vi "Compute Fit Curve v4.vi"(0 "X Array in":dbl[](array[numeric]), 1 "# Points":u32, 2 "Use Same Number of Points as Histogram":bool, 5 "Best Fit in":dbl[](array[numeric]), 7 "Y Array in":dbl[](array[numeric]), 11 "Error In":errorcluster, 12 "Fit Model":T2, 13 "Fit Parameters":variant, 14 "Ramp Type":T1 items=["Linear", "Logarithmic"]) -> (4 "Fitted Plot":cluster{"X Array":dbl[], "Y Array":dbl[]}, 6 "Array of Component Plots":cluster{"X Array":dbl[], "Y Array":dbl[]}[](array[cluster]), 8 "Residual Plot":cluster{"X Array":dbl[], "Y Array":dbl[]}, 15 "Error Out":errorcluster)   [LabVIEW 2019]
uses:
  Fit Models.ctl
  Ramp Type.ctl
  Gaussian Fit Results v2.ctl
  Two H-Connected Gaussians Fit Parameters.ctl
  Two H-Connected Asymmetric Gaussians Fit Parameters.ctl
  Asymmetric Gaussian Fit Results v2.ctl
  Two T-Connected Asymmetric Gaussians Fit Parameters.ctl
  Two T-Connected Gaussians Fit Parameters.ctl
  Asymmetric Lorentzian Fit Results v2.ctl
  Gaussian-Lorentzian Fit Results v2.ctl
  Lorentzian-Gaussian Fit Results v2.ctl
  Lorentzian Fit Results v2.ctl
  Single Exponential Fit Parameters v2.ctl
  Double Exponential Fit Parameters v2.ctl
  2D Gaussian ACF Fit Results.ctl
  2D Gaussian + Blinking ACF Fit Results.ctl
  2D Gaussian + Flow ACF Fit Results.ctl
  3D Gaussian ACF Fit Results.ctl
  3D Gaussian + Blinking ACF Fit Results.ctl
  <vilib>/Analysis/NI_AALBase.lvlib
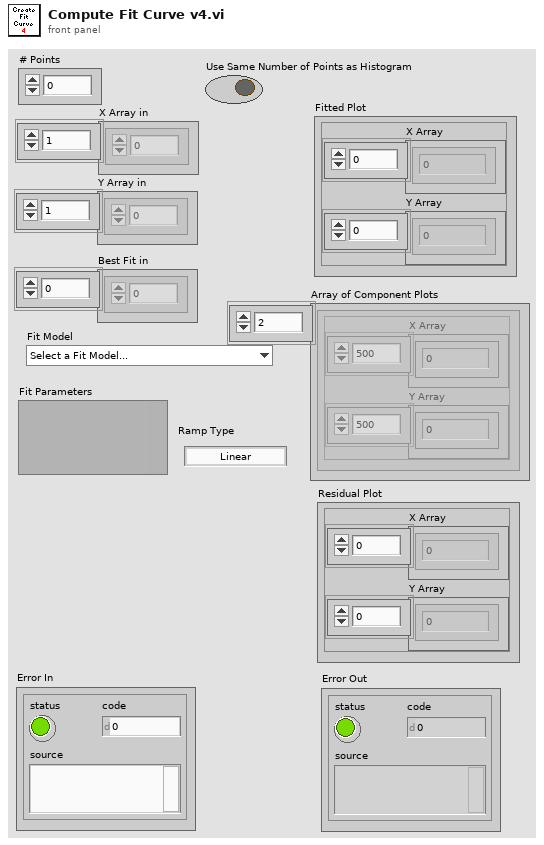
[diagram p1: front panel]
types:
  T1 = typedef "Ramp Type.ctl" = u16
  T2 = typedef "Fit Models.ctl" = enum16{"Select a Fit Model...", "           Single Peak", "Gaussian", "Asymmetric Gaussian", "Lorentzian", "Asymmetric Lorentzian", "Gaussian/Lorentzian", "Lorentzian/Gaussian", "           Double Peak", "Two Gaussians", "Two Asymmetric Gaussians", "Two H-Connected Gaussians", "Two T-Connected Gaussians", "Two H-Connected Asymmetric Gaussians", "Two T-Connected Asymmetric Gaussians", "           Triple Peak", "Three Gaussians", "Three Asymmetric Gaussians", "              Decays", "Single Exponential", "Two Exponentials", "               ACF", "2D Gaussian ACF", "2D Gaussian + Blinking ACF", "2D Gaussian + Flow ACF", "3D Gaussian ACF", "3D Gaussian + Blinking ACF", "             Multiplot", "2D Gaussian ACF & 2D Gaussian + Flow ACF"}
  T3 = typedef "Gaussian Fit Results v2.ctl" = cluster{"Amplitude":dbl, "Peak":dbl, "SDV":dbl, "FWHM":dbl, "Integral":dbl, "RMSE":dbl, "R^2":dbl}
  T4 = typedef "Two H-Connected Gaussians Fit Parameters.ctl" = cluster{"Gaussian Parameters":T3[], "Bridge Amplitude ":dbl}
  T5 = typedef "Two H-Connected Asymmetric Gaussians Fit Parameters.ctl" = cluster{"Asymmetric Gaussian Parameters":T6[], "Bridge Amplitude":dbl}
  T6 = typedef "Asymmetric Gaussian Fit Results v2.ctl" = cluster{"Amplitude":dbl, "Peak":dbl, "SDV-":dbl, "SDV+":dbl, "Mean":dbl, "SDV":dbl, "FWHM":dbl, "Integral":dbl, "RMSE":dbl, "R^2":dbl}
  T7 = typedef "Two T-Connected Asymmetric Gaussians Fit Parameters.ctl" = cluster{"Asymmetric Gaussian Parameters":T6[], "Bridge Amplitude":dbl, "Bridge Slope":dbl}
  T8 = typedef "Two T-Connected Gaussians Fit Parameters.ctl" = cluster{"Gaussian Parameters":T3[], "Bridge Amplitude ":dbl, "Bridge Slope":dbl}
  T9 = typedef "Asymmetric Lorentzian Fit Results v2.ctl" = cluster{"Amplitude":dbl, "Peak":dbl, "FWHM-":dbl, "FWHM+":dbl, "Integral":dbl, "RMSE":dbl, "R^2":dbl}
  T10 = typedef "Gaussian-Lorentzian Fit Results v2.ctl" = cluster{"Amplitude":dbl, "Peak":dbl, "SDV-":dbl, "FWHM+":dbl, "Mean":dbl, "FWHM":dbl, "Integral":dbl, " RMSE":dbl, "R^2":dbl}
  T11 = typedef "Lorentzian-Gaussian Fit Results v2.ctl" = cluster{"Amplitude":dbl, "Peak":dbl, "FWHM-":dbl, "SDV+":dbl, "Mean":dbl, "FWHM":dbl, "Integral":dbl, "RMSE":dbl, "R^2":dbl}
  T12 = typedef "Lorentzian Fit Results v2.ctl" = cluster{"Amplitude":dbl, "Peak":dbl, "FWHM":dbl, "Integral":dbl, "RMSE":dbl, "R^2":dbl}
  T13 = typedef "Single Exponential Fit Parameters v2.ctl" = cluster{"Amplitude":dbl, "Time Constant":dbl, "Mean":dbl, "SDV":dbl, "FWHM":dbl, "Integral":dbl, "MSE":dbl, "R^2":dbl}
  T14 = typedef "Double Exponential Fit Parameters v2.ctl" = cluster{"A1":dbl, "tau1":dbl, "A2":dbl, "tau2":dbl, "Mean":dbl, "SDV":dbl, "Integral":dbl, "MSE":dbl, "R^2":dbl}
  T15 = typedef "2D Gaussian ACF Fit Results.ctl" = cluster{"Amplitude":dbl, "Diffusion Time":dbl, "RMSE":dbl, "R^2":dbl}
  T16 = typedef "2D Gaussian + Blinking ACF Fit Results.ctl" = cluster{"Amplitude":dbl, "Diffusion Time":dbl, "Blinking Fraction":dbl, "Blinking Time Constant":dbl, "RMSE":dbl, "R^2":dbl}
  T17 = typedef "2D Gaussian + Flow ACF Fit Results.ctl" = cluster{"Amplitude":dbl, "Diffusion Time":dbl, "Translation Time":dbl, "RMSE":dbl, "R^2":dbl}
  T18 = typedef "3D Gaussian ACF Fit Results.ctl" = cluster{"Amplitude":dbl, "Diffusion Time":dbl, "Aspect Ratio":dbl, "RMSE":dbl, "R^2":dbl}
  T19 = typedef "3D Gaussian + Blinking ACF Fit Results.ctl" = cluster{"Amplitude":dbl, "Diffusion Time":dbl, "Aspect Ratio":dbl, "Blinking Fraction":dbl, "Blinking Time Constant":dbl, "RMSE":dbl, "R^2":dbl}
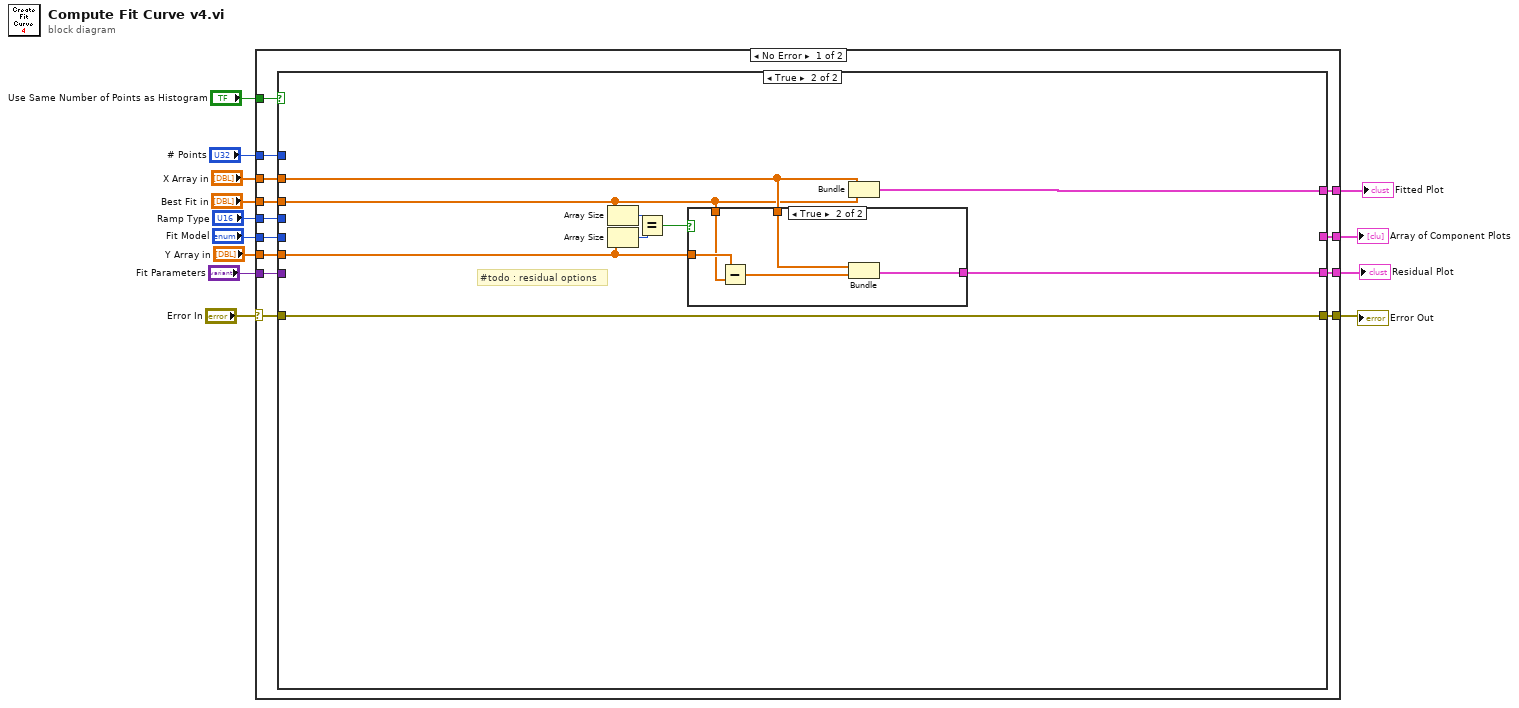
[diagram p0: block diagram]
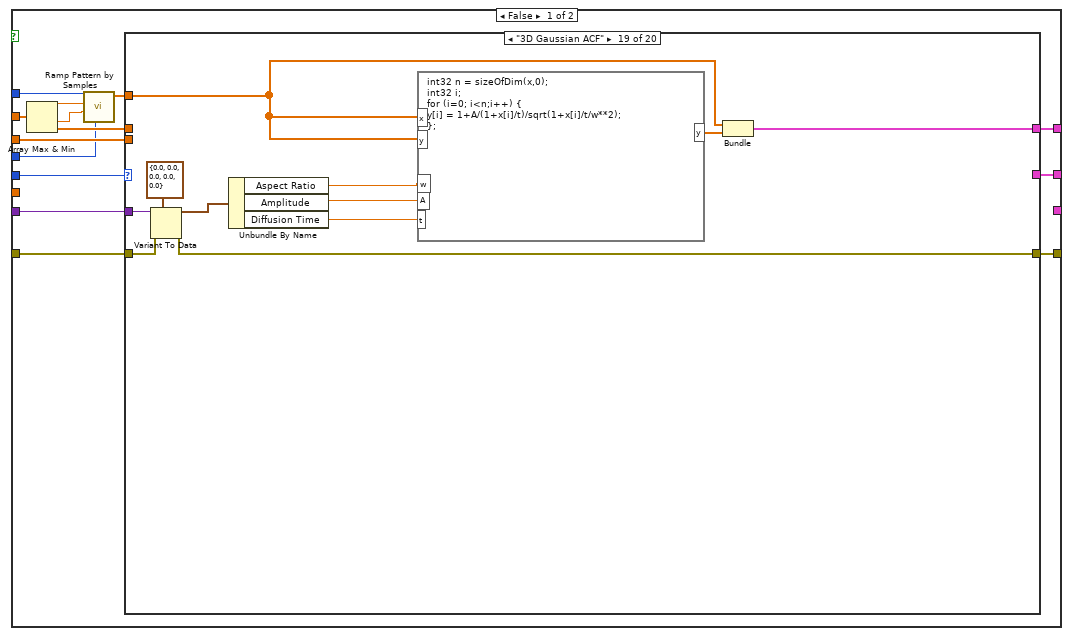
[diagram p2: hidden frame]
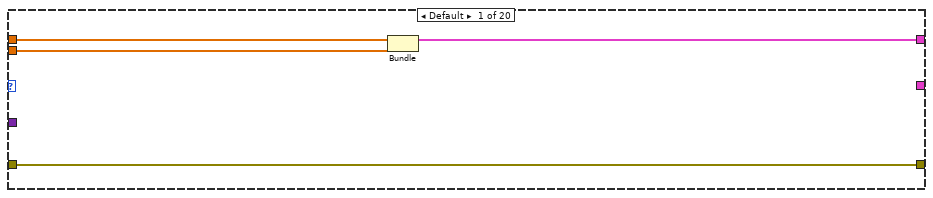
[diagram p3: hidden frame]
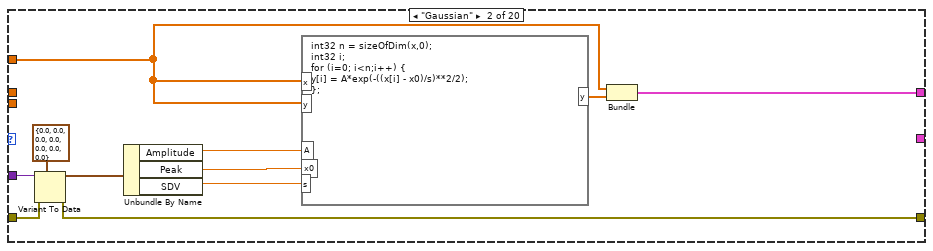
[diagram p4: hidden frame]
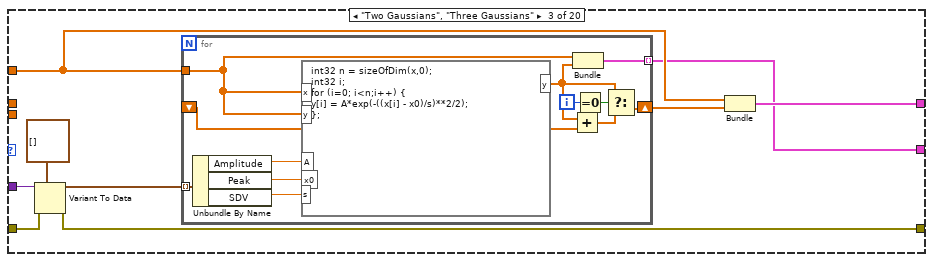
[diagram p5: hidden frame]
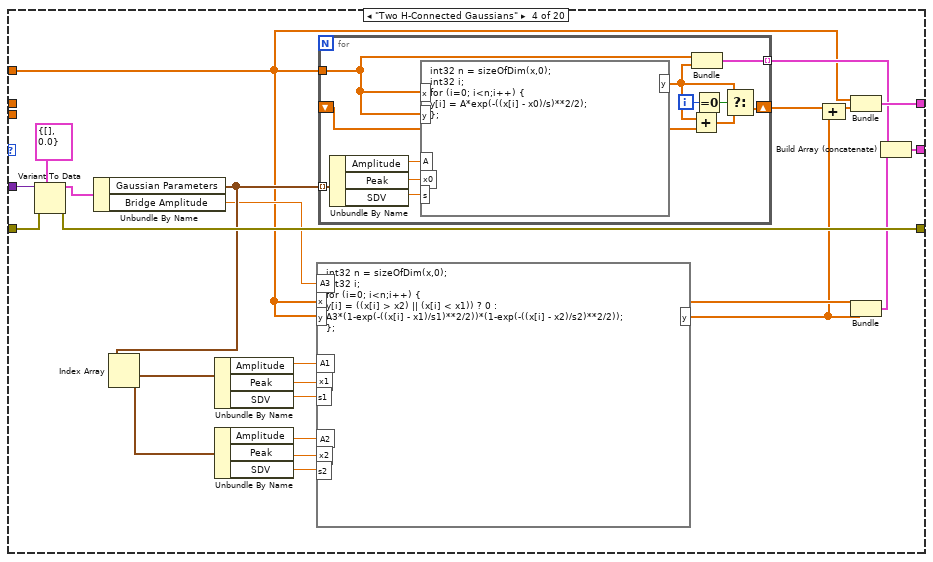
[diagram p6: hidden frame]
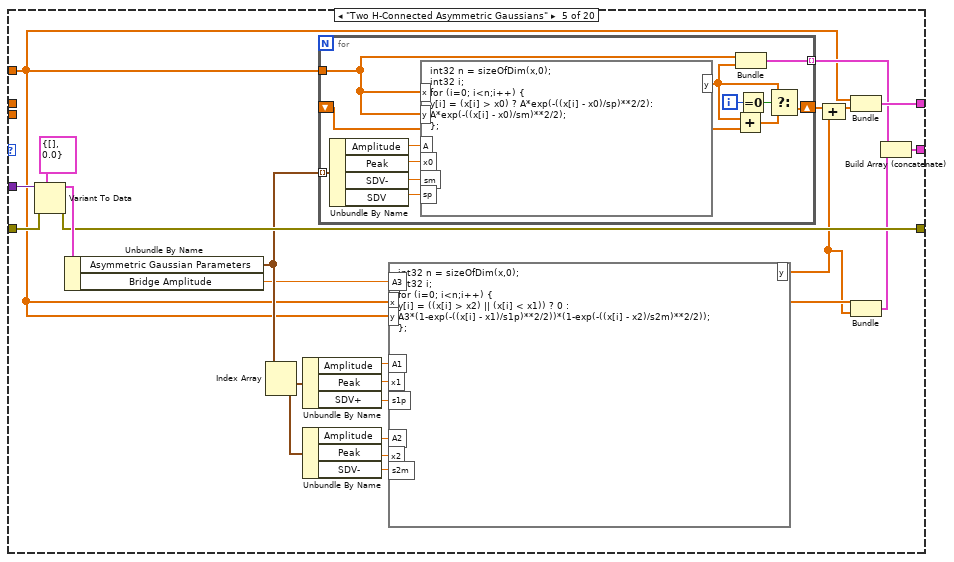
[diagram p7: hidden frame]
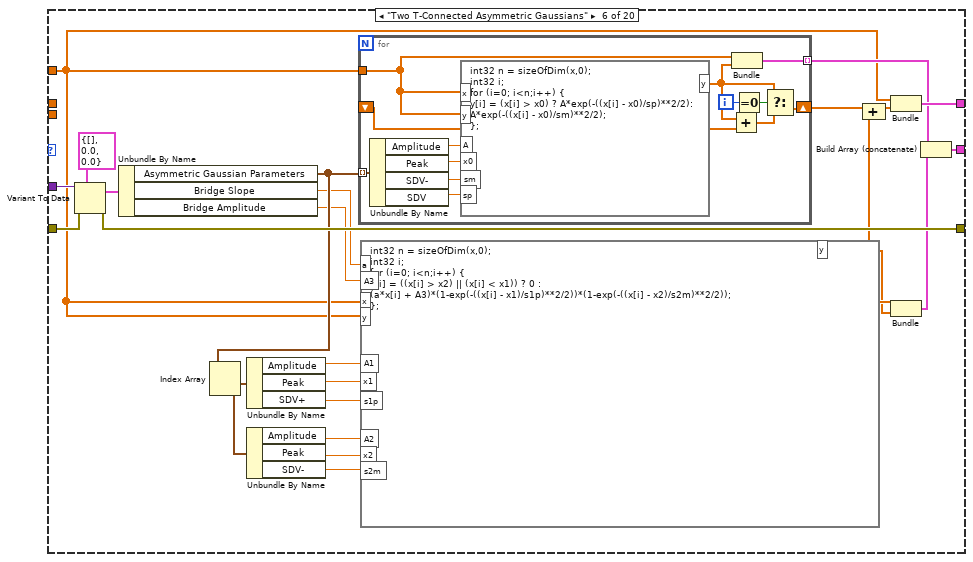
[diagram p8: hidden frame]
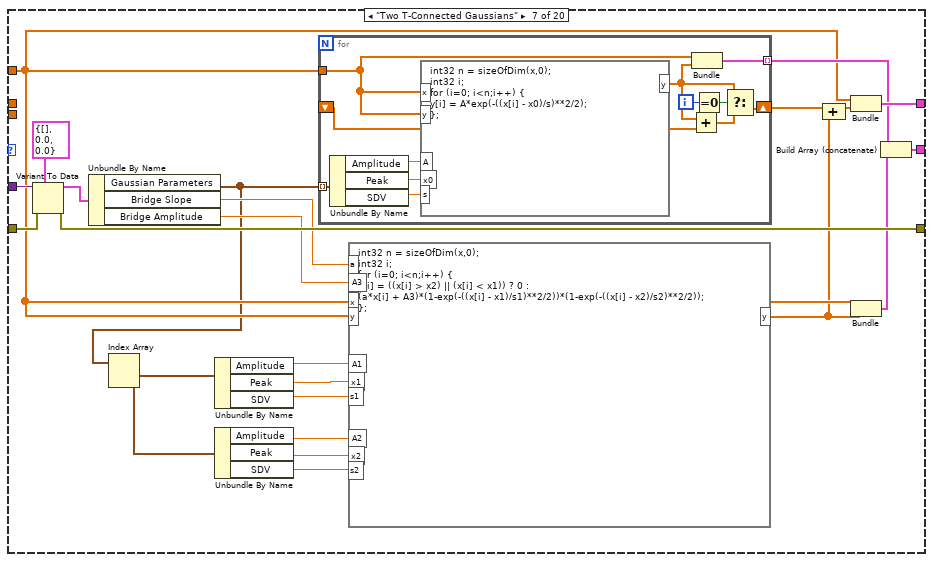
[diagram p9: hidden frame]
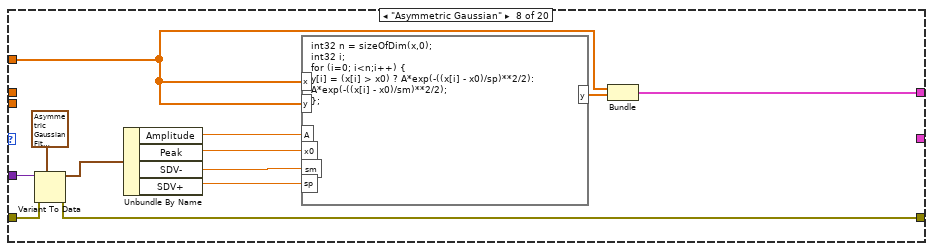
[diagram p10: hidden frame]
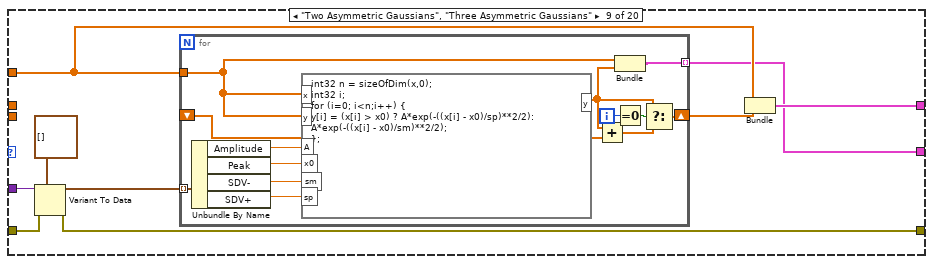
[diagram p11: hidden frame]
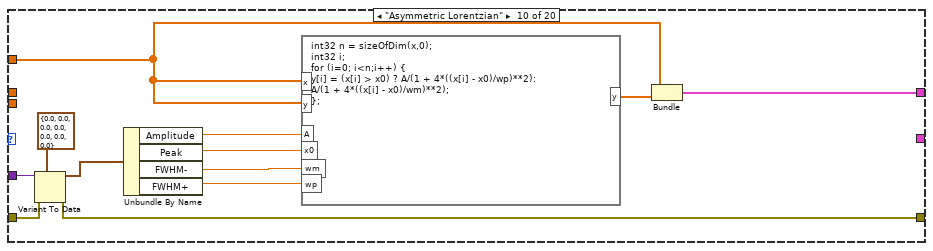
[diagram p12: hidden frame]
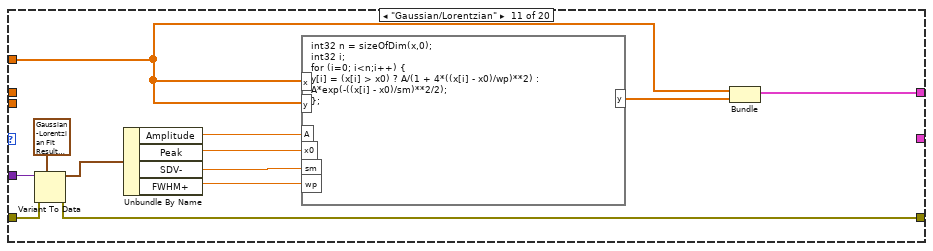
[diagram p13: hidden frame]
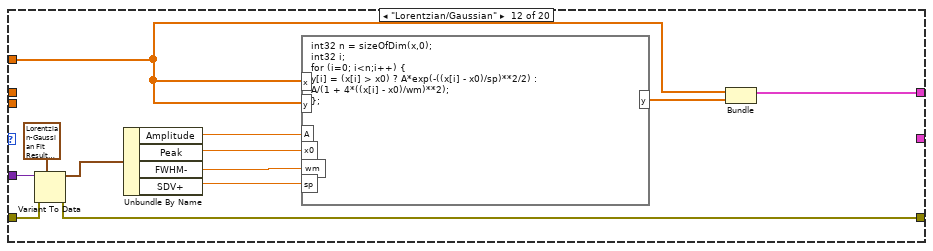
[diagram p14: hidden frame]
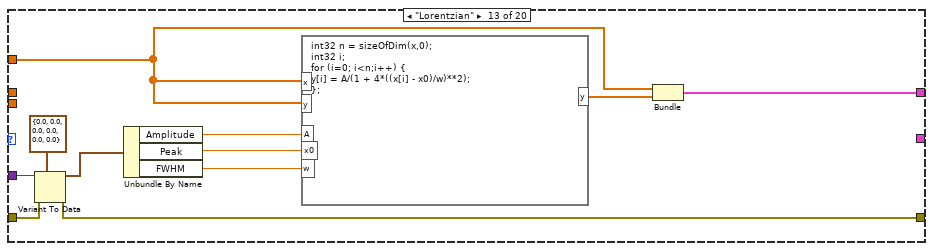
[diagram p15: hidden frame]
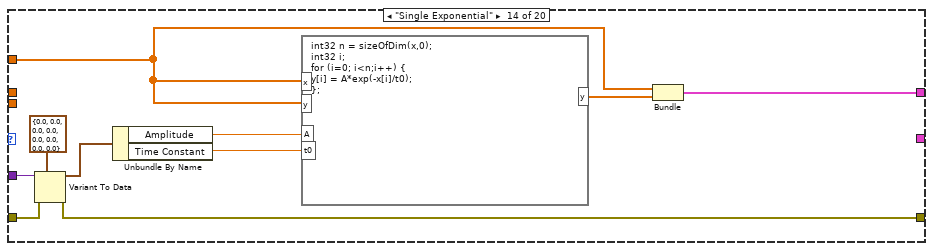
[diagram p16: hidden frame]
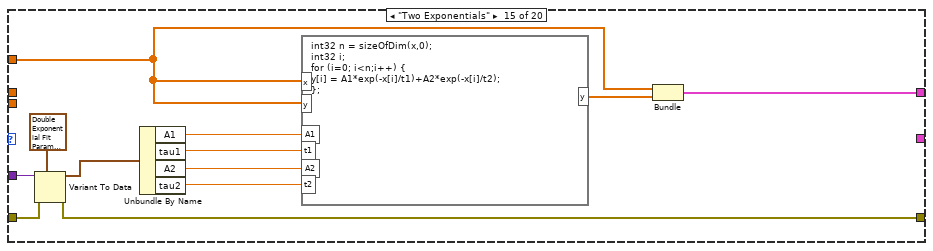
[diagram p17: hidden frame]
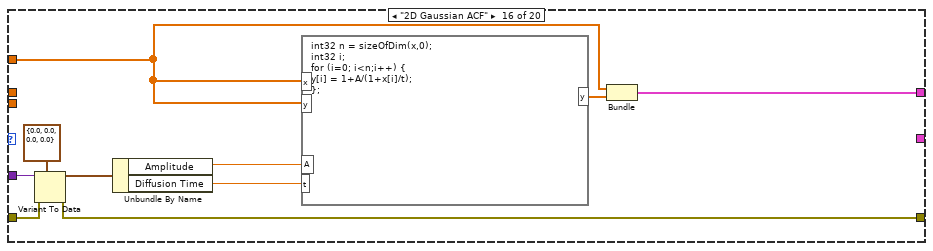
[diagram p18: hidden frame]
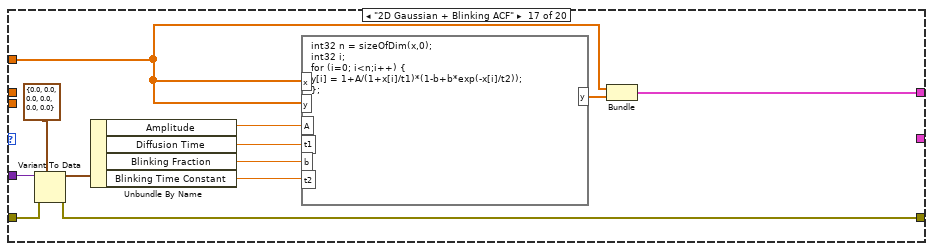
[diagram p19: hidden frame]
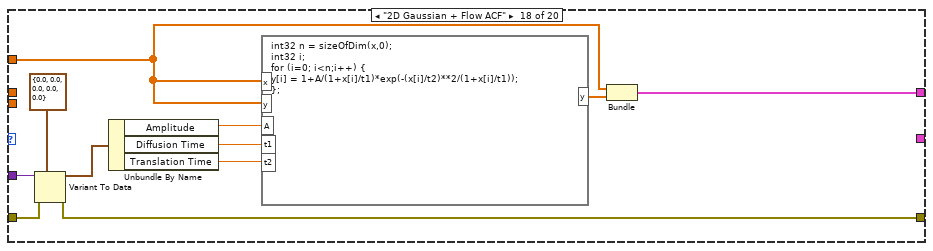
[diagram p20: hidden frame]
diagram:
  n1 = case shown="No Error" "Error In" {
    selector: "Error In" -> [w20 w397]
    tunnel: "Fit Model" -> [w26 _]
    tunnel: [w19 w397] -> w11
    tunnel: "Use Same Number of Points as Histogram" -> [w25 _]
    tunnel: "X Array in" -> [w24 w396]
    tunnel: "Best Fit in" -> [w23 w395]
    tunnel: "# Points" -> [w22 _]
    tunnel: "Fit Parameters" -> [w21 _]
    tunnel: [w17 _] -> w4
    tunnel: [w18 w394] -> w5
    tunnel: "Ramp Type" -> [w16 _]
    tunnel: [w15 _] -> w2
    tunnel: "Y Array in" -> [w14 _]
    frame No Error {
      n2 = case shown="True" w25 {
        tunnel: w26 -> [w39 _]
        tunnel: w24 -> [w32 w386]
        tunnel: w23 -> [w31 w383]
        tunnel: w22 -> [w38 _]
        tunnel: w21 -> [w34 _]
        tunnel: w20 -> [w33 w388]
        tunnel: [w30 w388] -> w19
        tunnel: [w29 w387] -> w18
        tunnel: [w28 _] -> w17
        tunnel: w16 -> [w27 _]
        tunnel: [_ w385] -> w15
        tunnel: w14 -> [_ w384]
        frame False {
          n3 = Array Max & Min(array=w32) -> (max value=w37:dbl, min value=w36:dbl)  [unwired: 2 out]
          n4 = call <vilib>:"Ramp Pattern by Samples.vi"("type"=w27, "start"=w36, "end"=w37, "samples"=w38) -> ("Ramp Pattern"=w35:dbl[])  [unwired: 6 in, 1 out]
          n5 = case shown="\"3D Gaussian ACF\"" w39 {
            tunnel: w35 -> [_ w44 w57 w80 w116 w153 w190 w221 w234 w255 w267 w278 w290 w302 w314 w323 w336 w347 w357 w371]
            tunnel: w34 -> [_ w54 w63 w98 w133 w170 w207 w231 w240 w265 w277 w289 w300 w310 w322 w332 w344 w355 w366 w379]
            tunnel: w33 -> [w43 w52 w62 w97 w132 w169 w206 w230 w239 w264 w276 w288 w299 w309 w321 w330 w343 w354 w364 w378]
            tunnel: w32 -> [w41 _ _ _ _ _ _ _ _ _ _ _ _ _ _ _ _ _ _ _]
            tunnel: w31 -> [w42 _ _ _ _ _ _ _ _ _ _ _ _ _ _ _ _ _ _ _]
            tunnel: [w43 w47 w60 w95 w130 w167 w204 w224 w237 w258 w270 w282 w294 w305 w317 w326 w339 w350 w360 w374] -> w30
            tunnel: [w40 w45 w56 w93 w128 w165 w202 w220 w233 w254 w266 w280 w292 w304 w316 w324 w337 w348 w358 w372] -> w29
            tunnel: [_ _ w55 w87 w122 w159 w197 _ w232 _ _ _ _ _ _ _ _ _ _ _] -> w28
            frame Default {
              n6 = Bundle("X Array in"=w41, "Best Fit in"=w42) -> (w40:cluster{"X Array in":dbl[], "Best Fit in":dbl[]})  [unwired: 1 in]
            }
            frame "Gaussian" {
              n7 = Variant To Data(error in=w52, type=T3 {"Amplitude"=0.0, "Peak"=0.0, "SDV"=0.0, "FWHM"=0.0, "Integral"=0.0, "RMSE"=0.0, "R^2"=0.0} ("Gaussian Fit Parameters"), Variant=w54) -> (data=w51:T3, error out=w47:errorcluster)
              n8 = Unbundle By Name(w51) -> ("Amplitude"=w50:dbl, "Peak"=w49:dbl, "SDV"=w48:dbl)
              n9 = formula code="int32 n = sizeOfDim(x,0);\nint32 i;\nfor (i=0; i<n;i++) {\ny[i] = A*exp(-((x[i] - x0)/s)**2/2);\n};"("A"=w50, "x0"=w49, "s"=w48, "x"=w44, "y"=w44) -> ("y"=w46:dbl[])
              n10 = Bundle("Ramp Pattern"=w44, "y"=w46) -> (w45:cluster{"Ramp Pattern":dbl[], "y":dbl[]})  [unwired: 1 in]
            }
            frame "Two Gaussians", "Three Gaussians" {
              n11 = Variant To Data(error in=w62, type=T3[] [] ("Two Gaussians Fit Parameters"), Variant=w63) -> (data=w61:T3[], error out=w60:errorcluster)
              n12 = for {
                tunnel: w61 -> [w75] mode=indexing
                tunnel: w57 -> [w65]
                shift-right: [w68] -> w58
                shift-left: _ -> [w69]
                tunnel: [w64] -> w55 mode=indexing
                i -> [w71]
                n13 = Unbundle By Name(w75) -> ("Amplitude"=w74:dbl, "Peak"=w73:dbl, "SDV"=w72:dbl)
                n14 = formula code="int32 n = sizeOfDim(x,0);\nint32 i;\nfor (i=0; i<n;i++) {\ny[i] = A*exp(-((x[i] - x0)/s)**2/2);\n};"("A"=w74, "x0"=w73, "s"=w72, "x"=w65, "y"=w65) -> ("y"=w66:dbl[])
                n15 = Add(x=w66, y=w69) -> (x+y=w67:dbl[])
                n16 = Bundle("Ramp Pattern"=w65, "y"=w66) -> (w64:cluster{"Ramp Pattern":dbl[], "y":dbl[]})  [unwired: 1 in]
                n17 = Equal To 0?(x=w71) -> (x = 0?=w70:bool)
                n18 = Select(t=w66, s=w70, f=w67) -> (s? t:f=w68:dbl[])
              }
              n19 = Bundle("Ramp Pattern"=w57, "y"=w58) -> (w56:cluster{"Ramp Pattern":dbl[], "y":dbl[]})  [unwired: 1 in]
            }
            frame "Two H-Connected Gaussians" {
              n20 = Variant To Data(error in=w97, type=T4 {"Gaussian Parameters"=[], "Bridge Amplitude "=0.0} ("Bridged Gaussians Parameters"), Variant=w98) -> (data=w96:T4, error out=w95:errorcluster)
              n21 = Unbundle By Name(w96) -> ("Gaussian Parameters"=w91:T3[], "Bridge Amplitude"=w88:dbl)
              n22 = Index Array(array=w91) -> (element #1=w90:T3, element #2=w89:T3)  [unwired: 2 in]
              n23 = Unbundle By Name(w90) -> ("Amplitude"=w86:dbl, "Peak"=w85:dbl, "SDV"=w84:dbl)
              n24 = Unbundle By Name(w89) -> ("Amplitude"=w81:dbl, "Peak"=w82:dbl, "SDV"=w83:dbl)
              n25 = formula code="int32 n = sizeOfDim(x,0);\nint32 i;\nfor (i=0; i<n;i++) {\ny[i] = ((x[i] > x2) || (x[i] < x1)) ? 0 : \nA3*(1-exp(-((x[i] - x1)/s1)**2/2))*(1-exp(-((x[i] - x2)/s2)**2/2));\n};"("A1"=w86, "x1"=w85, "s1"=w84, "x"=w80, "y"=w80, "A2"=w81, "x2"=w82, "s2"=w83, "A3"=w88) -> ("y"=w77:dbl[])
              n26 = for {
                tunnel: w91 -> [w110] mode=indexing
                tunnel: w80 -> [w100]
                shift-right: [w103] -> w94
                shift-left: _ -> [w104]
                tunnel: [w99] -> w92 mode=indexing
                i -> [w106]
                n27 = Unbundle By Name(w110) -> ("Amplitude"=w109:dbl, "Peak"=w108:dbl, "SDV"=w107:dbl)
                n28 = formula code="int32 n = sizeOfDim(x,0);\nint32 i;\nfor (i=0; i<n;i++) {\ny[i] = A*exp(-((x[i] - x0)/s)**2/2);\n};"("A"=w109, "x0"=w108, "s"=w107, "x"=w100, "y"=w100) -> ("y"=w101:dbl[])
                n29 = Add(x=w101, y=w104) -> (x+y=w102:dbl[])
                n30 = Bundle("Ramp Pattern"=w100, "y"=w101) -> (w99:cluster{"Ramp Pattern":dbl[], "y":dbl[]})  [unwired: 1 in]
                n31 = Equal To 0?(x=w106) -> (x = 0?=w105:bool)
                n32 = Select(t=w101, s=w105, f=w102) -> (s? t:f=w103:dbl[])
              }
              n33 = Compound Arithmetic op=ADD(w94, w77) -> (w78:dbl[])
              n34 = Bundle("Ramp Pattern"=w80, w78) -> (w93:cluster{"Ramp Pattern":dbl[], dbl[]})  [unwired: 1 in]
              n35 = Bundle("Ramp Pattern"=w80, "y"=w77) -> (w79:cluster{"Ramp Pattern":dbl[], "y":dbl[]})  [unwired: 1 in]
              n36 = Build Array (concatenate)(w92, w79) -> (w87:cluster{"Ramp Pattern":dbl[], "y":dbl[]}[])
            }
            frame "Two H-Connected Asymmetric Gaussians" {
              n37 = Variant To Data(error in=w132, type=T5 {"Asymmetric Gaussian Parameters"=[], "Bridge Amplitude"=0.0} ("output cluster"), Variant=w133) -> (data=w131:T5, error out=w130:errorcluster)
              n38 = Unbundle By Name(w131) -> ("Asymmetric Gaussian Parameters"=w126:T6[], "Bridge Amplitude"=w123:dbl)
              n39 = Index Array(array=w126) -> (element #1=w125:T6, element #2=w124:T6)  [unwired: 2 in]
              n40 = Unbundle By Name(w125) -> ("Amplitude"=w121:dbl, "Peak"=w120:dbl, "SDV+"=w112:dbl)
              n41 = Unbundle By Name(w124) -> ("Amplitude"=w117:dbl, "Peak"=w118:dbl, "SDV-"=w119:dbl)
              n42 = for {
                tunnel: w126 -> [w146] mode=indexing
                tunnel: w116 -> [w135]
                shift-right: [w138] -> w129
                shift-left: _ -> [w139]
                tunnel: [w134] -> w127 mode=indexing
                i -> [w141]
                n43 = Unbundle By Name(w146) -> ("Amplitude"=w145:dbl, "Peak"=w144:dbl, "SDV-"=w143:dbl, "SDV"=w142:dbl)
                n44 = formula code="int32 n = sizeOfDim(x,0);\nint32 i;\nfor (i=0; i<n;i++) {\ny[i] = (x[i] > x0) ? A*exp(-((x[i] - x0)/sp)**2/2):\nA*exp(-((x[i] - x0)/sm)**2/2);\n};"("A"=w145, "x0"=w144, "sm"=w143, "sp"=w142, "x"=w135, "y"=w135) -> ("y"=w136:dbl[])
                n45 = Add(x=w136, y=w139) -> (x+y=w137:dbl[])
                n46 = Bundle("Ramp Pattern"=w135, "y"=w136) -> (w134:cluster{"Ramp Pattern":dbl[], "y":dbl[]})  [unwired: 1 in]
                n47 = Equal To 0?(x=w141) -> (x = 0?=w140:bool)
                n48 = Select(t=w136, s=w140, f=w137) -> (s? t:f=w138:dbl[])
              }
              n49 = formula code="int32 n = sizeOfDim(x,0);\nint32 i;\nfor (i=0; i<n;i++) {\ny[i] = ((x[i] > x2) || (x[i] < x1)) ? 0 : \nA3*(1-exp(-((x[i] - x1)/s1p)**2/2))*(1-exp(-((x[i] - x2)/s2m)**2/2));\n};"("A1"=w121, "x1"=w120, "x"=w116, "y"=w116, "A2"=w117, "x2"=w118, "s2m"=w119, "A3"=w123, "s1p"=w112) -> ("y"=w113:dbl[])
              n50 = Compound Arithmetic op=ADD(w129, w113) -> (w114:dbl[])
              n51 = Bundle("Ramp Pattern"=w116, w114) -> (w128:cluster{"Ramp Pattern":dbl[], dbl[]})  [unwired: 1 in]
              n52 = Bundle("Ramp Pattern"=w116, "y"=w113) -> (w115:cluster{"Ramp Pattern":dbl[], "y":dbl[]})  [unwired: 1 in]
              n53 = Build Array (concatenate)(w127, w115) -> (w122:cluster{"Ramp Pattern":dbl[], "y":dbl[]}[])
            }
            frame "Two T-Connected Asymmetric Gaussians" {
              n54 = Variant To Data(error in=w169, type=T7 {"Asymmetric Gaussian Parameters"=[], "Bridge Amplitude"=0.0, "Bridge Slope"=0.0} ("Two T-Connected Asymmetric Gaussian Parameters"), Variant=w170) -> (data=w168:T7, error out=w167:errorcluster)
              n55 = Unbundle By Name(w168) -> ("Asymmetric Gaussian Parameters"=w163:T6[], "Bridge Slope"=w160:dbl, "Bridge Amplitude"=w148:dbl)
              n56 = Index Array(array=w163) -> (element #1=w162:T6, element #2=w161:T6)  [unwired: 2 in]
              n57 = Unbundle By Name(w162) -> ("Amplitude"=w158:dbl, "Peak"=w157:dbl, "SDV+"=w149:dbl)
              n58 = Unbundle By Name(w161) -> ("Amplitude"=w154:dbl, "Peak"=w155:dbl, "SDV-"=w156:dbl)
              n59 = for {
                tunnel: w163 -> [w183] mode=indexing
                tunnel: w153 -> [w172]
                shift-right: [w175] -> w166
                shift-left: _ -> [w176]
                tunnel: [w171] -> w164 mode=indexing
                i -> [w178]
                n60 = Unbundle By Name(w183) -> ("Amplitude"=w182:dbl, "Peak"=w181:dbl, "SDV-"=w180:dbl, "SDV"=w179:dbl)
                n61 = formula code="int32 n = sizeOfDim(x,0);\nint32 i;\nfor (i=0; i<n;i++) {\ny[i] = (x[i] > x0) ? A*exp(-((x[i] - x0)/sp)**2/2):\nA*exp(-((x[i] - x0)/sm)**2/2);\n};"("A"=w182, "x0"=w181, "sm"=w180, "sp"=w179, "x"=w172, "y"=w172) -> ("y"=w173:dbl[])
                n62 = Add(x=w173, y=w176) -> (x+y=w174:dbl[])
                n63 = Bundle("Ramp Pattern"=w172, "y"=w173) -> (w171:cluster{"Ramp Pattern":dbl[], "y":dbl[]})  [unwired: 1 in]
                n64 = Equal To 0?(x=w178) -> (x = 0?=w177:bool)
                n65 = Select(t=w173, s=w177, f=w174) -> (s? t:f=w175:dbl[])
              }
              n66 = formula code="int32 n = sizeOfDim(x,0);\nint32 i;\nfor (i=0; i<n;i++) {\ny[i] = ((x[i] > x2) || (x[i] < x1)) ? 0 : \n(a*x[i] + A3)*(1-exp(-((x[i] - x1)/s1p)**2/2))*(1-exp(-((x[i] - x2)/s2m)**2/2));\n};"("A1"=w158, "x1"=w157, "x"=w153, "y"=w153, "A2"=w154, "x2"=w155, "s2m"=w156, "a"=w160, "s1p"=w149, "A3"=w148) -> ("y"=w150:dbl[])
              n67 = Compound Arithmetic op=ADD(w166, w150) -> (w151:dbl[])
              n68 = Bundle("Ramp Pattern"=w153, w151) -> (w165:cluster{"Ramp Pattern":dbl[], dbl[]})  [unwired: 1 in]
              n69 = Bundle("Ramp Pattern"=w153, "y"=w150) -> (w152:cluster{"Ramp Pattern":dbl[], "y":dbl[]})  [unwired: 1 in]
              n70 = Build Array (concatenate)(w164, w152) -> (w159:cluster{"Ramp Pattern":dbl[], "y":dbl[]}[])
            }
            frame "Two T-Connected Gaussians" {
              n71 = Variant To Data(error in=w206, type=T8 {"Gaussian Parameters"=[], "Bridge Amplitude "=0.0, "Bridge Slope"=0.0} ("Bridged Gaussians Parameters"), Variant=w207) -> (data=w205:T8, error out=w204:errorcluster)
              n72 = Unbundle By Name(w205) -> ("Gaussian Parameters"=w184:T3[], "Bridge Slope"=w198:dbl, "Bridge Amplitude"=w186:dbl)
              n73 = Index Array(array=w184) -> (element #1=w200:T3, element #2=w199:T3)  [unwired: 2 in]
              n74 = Unbundle By Name(w200) -> ("Amplitude"=w196:dbl, "Peak"=w195:dbl, "SDV"=w194:dbl)
              n75 = Unbundle By Name(w199) -> ("Amplitude"=w191:dbl, "Peak"=w192:dbl, "SDV"=w193:dbl)
              n76 = for {
                tunnel: w184 -> [w219] mode=indexing
                tunnel: w190 -> [w209]
                shift-right: [w212] -> w203
                shift-left: _ -> [w213]
                tunnel: [w208] -> w201 mode=indexing
                i -> [w215]
                n77 = Unbundle By Name(w219) -> ("Amplitude"=w218:dbl, "Peak"=w217:dbl, "SDV"=w216:dbl)
                n78 = formula code="int32 n = sizeOfDim(x,0);\nint32 i;\nfor (i=0; i<n;i++) {\ny[i] = A*exp(-((x[i] - x0)/s)**2/2);\n};"("A"=w218, "x0"=w217, "s"=w216, "x"=w209, "y"=w209) -> ("y"=w210:dbl[])
                n79 = Add(x=w210, y=w213) -> (x+y=w211:dbl[])
                n80 = Bundle("Ramp Pattern"=w209, "y"=w210) -> (w208:cluster{"Ramp Pattern":dbl[], "y":dbl[]})  [unwired: 1 in]
                n81 = Equal To 0?(x=w215) -> (x = 0?=w214:bool)
                n82 = Select(t=w210, s=w214, f=w211) -> (s? t:f=w212:dbl[])
              }
              n83 = formula code="int32 n = sizeOfDim(x,0);\nint32 i;\nfor (i=0; i<n;i++) {\ny[i] = ((x[i] > x2) || (x[i] < x1)) ? 0 : \n(a*x[i] + A3)*(1-exp(-((x[i] - x1)/s1)**2/2))*(1-exp(-((x[i] - x2)/s2)**2/2));\n};"("A1"=w196, "x1"=w195, "s1"=w194, "x"=w190, "y"=w190, "A2"=w191, "x2"=w192, "s2"=w193, "a"=w198, "A3"=w186) -> ("y"=w187:dbl[])
              n84 = Compound Arithmetic op=ADD(w203, w187) -> (w188:dbl[])
              n85 = Bundle("Ramp Pattern"=w190, w188) -> (w202:cluster{"Ramp Pattern":dbl[], dbl[]})  [unwired: 1 in]
              n86 = Bundle("Ramp Pattern"=w190, "y"=w187) -> (w189:cluster{"Ramp Pattern":dbl[], "y":dbl[]})  [unwired: 1 in]
              n87 = Build Array (concatenate)(w201, w189) -> (w197:cluster{"Ramp Pattern":dbl[], "y":dbl[]}[])
            }
            frame "Asymmetric Gaussian" {
              n88 = Variant To Data(error in=w230, type=T6 {"Amplitude"=0.0, "Peak"=0.0, "SDV-"=0.0, "SDV+"=0.0, "Mean"=0.0, "SDV"=0.0, "FWHM"=0.0, "Integral"=0.0, "RMSE"=0.0, "R^2"=0.0} ("Asymmetric Gaussian Fit Parameters"), Variant=w231) -> (data=w229:T6, error out=w224:errorcluster)
              n89 = Unbundle By Name(w229) -> ("Amplitude"=w228:dbl, "Peak"=w227:dbl, "SDV-"=w226:dbl, "SDV+"=w225:dbl)
              n90 = formula code="int32 n = sizeOfDim(x,0);\nint32 i;\nfor (i=0; i<n;i++) {\ny[i] = (x[i] > x0) ? A*exp(-((x[i] - x0)/sp)**2/2):\nA*exp(-((x[i] - x0)/sm)**2/2);\n};"("A"=w228, "x0"=w227, "sm"=w226, "sp"=w225, "x"=w221, "y"=w221) -> ("y"=w222:dbl[])
              n91 = Bundle("Ramp Pattern"=w221, "y"=w222) -> (w220:cluster{"Ramp Pattern":dbl[], "y":dbl[]})  [unwired: 1 in]
            }
            frame "Two Asymmetric Gaussians", "Three Asymmetric Gaussians" {
              n92 = Variant To Data(error in=w239, type=T6[] [] ("Two Asymmetric Gaussians Fit Parameters"), Variant=w240) -> (data=w238:T6[], error out=w237:errorcluster)
              n93 = for {
                tunnel: w238 -> [w253] mode=indexing
                tunnel: w234 -> [w242]
                shift-right: [w246] -> w235
                shift-left: _ -> [w245]
                tunnel: [w241] -> w232 mode=indexing
                i -> [w247]
                n94 = Unbundle By Name(w253) -> ("Amplitude"=w252:dbl, "Peak"=w251:dbl, "SDV-"=w250:dbl, "SDV+"=w249:dbl)
                n95 = formula code="int32 n = sizeOfDim(x,0);\nint32 i;\nfor (i=0; i<n;i++) {\ny[i] = (x[i] > x0) ? A*exp(-((x[i] - x0)/sp)**2/2):\nA*exp(-((x[i] - x0)/sm)**2/2);\n};"("A"=w252, "x0"=w251, "sm"=w250, "sp"=w249, "x"=w242, "y"=w242) -> ("y"=w243:dbl[])
                n96 = Add(x=w243, y=w245) -> (x+y=w244:dbl[])
                n97 = Bundle("Ramp Pattern"=w242, "y"=w243) -> (w241:cluster{"Ramp Pattern":dbl[], "y":dbl[]})  [unwired: 1 in]
                n98 = Equal To 0?(x=w247) -> (x = 0?=w248:bool)
                n99 = Select(t=w243, s=w248, f=w244) -> (s? t:f=w246:dbl[])
              }
              n100 = Bundle("Ramp Pattern"=w234, "y"=w235) -> (w233:cluster{"Ramp Pattern":dbl[], "y":dbl[]})  [unwired: 1 in]
            }
            frame "Asymmetric Lorentzian" {
              n101 = Variant To Data(error in=w264, type=T9 {"Amplitude"=0.0, "Peak"=0.0, "FWHM-"=0.0, "FWHM+"=0.0, "Integral"=0.0, "RMSE"=0.0, "R^2"=0.0} ("Asymmetric Lorentz Fit Parameters"), Variant=w265) -> (data=w263:T9, error out=w258:errorcluster)
              n102 = Unbundle By Name(w263) -> ("Amplitude"=w262:dbl, "Peak"=w261:dbl, "FWHM-"=w260:dbl, "FWHM+"=w259:dbl)
              n103 = formula code="int32 n = sizeOfDim(x,0);\nint32 i;\nfor (i=0; i<n;i++) {\ny[i] = (x[i] > x0) ? A/(1 + 4*((x[i] - x0)/wp)**2):\nA/(1 + 4*((x[i] - x0)/wm)**2);\n};"("A"=w262, "x0"=w261, "wm"=w260, "wp"=w259, "x"=w255, "y"=w255) -> ("y"=w256:dbl[])
              n104 = Bundle("Ramp Pattern"=w255, "y"=w256) -> (w254:cluster{"Ramp Pattern":dbl[], "y":dbl[]})  [unwired: 1 in]
            }
            frame "Gaussian/Lorentzian" {
              n105 = Variant To Data(error in=w276, type=T10 {"Amplitude"=0.0, "Peak"=0.0, "SDV-"=0.0, "FWHM+"=0.0, "Mean"=0.0, "FWHM"=0.0, "Integral"=0.0, " RMSE"=0.0, "R^2"=0.0} ("Gaussian/Lorentzian Fit Parameters"), Variant=w277) -> (data=w275:T10, error out=w270:errorcluster)
              n106 = Unbundle By Name(w275) -> ("Amplitude"=w274:dbl, "Peak"=w273:dbl, "SDV-"=w272:dbl, "FWHM+"=w271:dbl)
              n107 = formula code="int32 n = sizeOfDim(x,0);\nint32 i;\nfor (i=0; i<n;i++) {\ny[i] = (x[i] > x0) ? A/(1 + 4*((x[i] - x0)/wp)**2) :\nA*exp(-((x[i] - x0)/sm)**2/2);\n};"("A"=w274, "x0"=w273, "sm"=w272, "wp"=w271, "x"=w267, "y"=w267) -> ("y"=w268:dbl[])
              n108 = Bundle("Ramp Pattern"=w267, "y"=w268) -> (w266:cluster{"Ramp Pattern":dbl[], "y":dbl[]})  [unwired: 1 in]
            }
            frame "Lorentzian/Gaussian" {
              n109 = Variant To Data(error in=w288, type=T11 {"Amplitude"=0.0, "Peak"=0.0, "FWHM-"=0.0, "SDV+"=0.0, "Mean"=0.0, "FWHM"=0.0, "Integral"=0.0, "RMSE"=0.0, "R^2"=0.0} ("Lorentzian/Gaussian Fit Parameters"), Variant=w289) -> (data=w287:T11, error out=w282:errorcluster)
              n110 = Unbundle By Name(w287) -> ("Amplitude"=w286:dbl, "Peak"=w285:dbl, "FWHM-"=w284:dbl, "SDV+"=w283:dbl)
              n111 = formula code="int32 n = sizeOfDim(x,0);\nint32 i;\nfor (i=0; i<n;i++) {\ny[i] = (x[i] > x0) ? A*exp(-((x[i] - x0)/sp)**2/2) :\nA/(1 + 4*((x[i] - x0)/wm)**2);\n};"("A"=w286, "x0"=w285, "wm"=w284, "sp"=w283, "x"=w278, "y"=w278) -> ("y"=w279:dbl[])
              n112 = Bundle("Ramp Pattern"=w278, "y"=w279) -> (w280:cluster{"Ramp Pattern":dbl[], "y":dbl[]})  [unwired: 1 in]
            }
            frame "Lorentzian" {
              n113 = Variant To Data(error in=w299, type=T12 {"Amplitude"=0.0, "Peak"=0.0, "FWHM"=0.0, "Integral"=0.0, "RMSE"=0.0, "R^2"=0.0} ("Lorentz Fit Parameters"), Variant=w300) -> (data=w298:T12, error out=w294:errorcluster)
              n114 = Unbundle By Name(w298) -> ("Amplitude"=w297:dbl, "Peak"=w296:dbl, "FWHM"=w295:dbl)
              n115 = formula code="int32 n = sizeOfDim(x,0);\nint32 i;\nfor (i=0; i<n;i++) {\ny[i] = A/(1 + 4*((x[i] - x0)/w)**2);\n};"("A"=w297, "x0"=w296, "w"=w295, "x"=w290, "y"=w290) -> ("y"=w291:dbl[])
              n116 = Bundle("Ramp Pattern"=w290, "y"=w291) -> (w292:cluster{"Ramp Pattern":dbl[], "y":dbl[]})  [unwired: 1 in]
            }
            frame "Single Exponential" {
              n117 = Variant To Data(error in=w309, type=T13 {"Amplitude"=0.0, "Time Constant"=0.0, "Mean"=0.0, "SDV"=0.0, "FWHM"=0.0, "Integral"=0.0, "MSE"=0.0, "R^2"=0.0} ("Single Exponential Fit Parameters"), Variant=w310) -> (data=w308:T13, error out=w305:errorcluster)
              n118 = Unbundle By Name(w308) -> ("Amplitude"=w307:dbl, "Time Constant"=w306:dbl)
              n119 = formula code="int32 n = sizeOfDim(x,0);\nint32 i;\nfor (i=0; i<n;i++) {\ny[i] = A*exp(-x[i]/t0);\n};"("A"=w307, "t0"=w306, "x"=w302, "y"=w302) -> ("y"=w303:dbl[])
              n120 = Bundle("Ramp Pattern"=w302, "y"=w303) -> (w304:cluster{"Ramp Pattern":dbl[], "y":dbl[]})  [unwired: 1 in]
            }
            frame "Two Exponentials" {
              n121 = Variant To Data(error in=w321, type=T14 {"A1"=0.0, "tau1"=0.0, "A2"=0.0, "tau2"=0.0, "Mean"=0.0, "SDV"=0.0, "Integral"=0.0, "MSE"=0.0, "R^2"=0.0} ("Double Exponential Fit Parameters"), Variant=w322) -> (data=w320:T14, error out=w317:errorcluster)
              n122 = Unbundle By Name(w320) -> ("A1"=w319:dbl, "tau1"=w318:dbl, "A2"=w312:dbl, "tau2"=w311:dbl)
              n123 = formula code="int32 n = sizeOfDim(x,0);\nint32 i;\nfor (i=0; i<n;i++) {\ny[i] = A1*exp(-x[i]/t1)+A2*exp(-x[i]/t2);\n};"("A1"=w319, "t1"=w318, "x"=w314, "y"=w314, "A2"=w312, "t2"=w311) -> ("y"=w315:dbl[])
              n124 = Bundle("Ramp Pattern"=w314, "y"=w315) -> (w316:cluster{"Ramp Pattern":dbl[], "y":dbl[]})  [unwired: 1 in]
            }
            frame "2D Gaussian ACF" {
              n125 = Variant To Data(error in=w330, type=T15 {"Amplitude"=0.0, "Diffusion Time"=0.0, "RMSE"=0.0, "R^2"=0.0} ("2D ACF Fit Parameters"), Variant=w332) -> (data=w329:T15, error out=w326:errorcluster)
              n126 = Unbundle By Name(w329) -> ("Amplitude"=w328:dbl, "Diffusion Time"=w327:dbl)
              n127 = formula code="int32 n = sizeOfDim(x,0);\nint32 i;\nfor (i=0; i<n;i++) {\ny[i] = 1+A/(1+x[i]/t);\n};"("A"=w328, "t"=w327, "x"=w323, "y"=w323) -> ("y"=w325:dbl[])
              n128 = Bundle("Ramp Pattern"=w323, "y"=w325) -> (w324:cluster{"Ramp Pattern":dbl[], "y":dbl[]})  [unwired: 1 in]
            }
            frame "2D Gaussian + Blinking ACF" {
              n129 = Variant To Data(error in=w343, type=T16 {"Amplitude"=0.0, "Diffusion Time"=0.0, "Blinking Fraction"=0.0, "Blinking Time Constant"=0.0, "RMSE"=0.0, "R^2"=0.0} ("2D Gaussian + Blinking ACF Fit Parameters"), Variant=w344) -> (data=w342:T16, error out=w339:errorcluster)
              n130 = Unbundle By Name(w342) -> ("Amplitude"=w341:dbl, "Diffusion Time"=w340:dbl, "Blinking Fraction"=w334:dbl, "Blinking Time Constant"=w333:dbl)
              n131 = formula code="int32 n = sizeOfDim(x,0);\nint32 i;\nfor (i=0; i<n;i++) {\ny[i] = 1+A/(1+x[i]/t1)*(1-b+b*exp(-x[i]/t2));\n};"("A"=w341, "t1"=w340, "x"=w336, "y"=w336, "b"=w334, "t2"=w333) -> ("y"=w338:dbl[])
              n132 = Bundle("Ramp Pattern"=w336, "y"=w338) -> (w337:cluster{"Ramp Pattern":dbl[], "y":dbl[]})  [unwired: 1 in]
            }
            frame "2D Gaussian + Flow ACF" {
              n133 = Variant To Data(error in=w354, type=T17 {"Amplitude"=0.0, "Diffusion Time"=0.0, "Translation Time"=0.0, "RMSE"=0.0, "R^2"=0.0} ("2D Gaussian + Blinking ACF Fit Parameters"), Variant=w355) -> (data=w353:T17, error out=w350:errorcluster)
              n134 = Unbundle By Name(w353) -> ("Amplitude"=w352:dbl, "Diffusion Time"=w351:dbl, "Translation Time"=w346:dbl)
              n135 = formula code="int32 n = sizeOfDim(x,0);\nint32 i;\nfor (i=0; i<n;i++) {\ny[i] = 1+A/(1+x[i]/t1)*exp(-(x[i]/t2)**2/(1+x[i]/t1));\n};"("A"=w352, "t1"=w351, "x"=w347, "y"=w347, "t2"=w346) -> ("y"=w349:dbl[])
              n136 = Bundle("Ramp Pattern"=w347, "y"=w349) -> (w348:cluster{"Ramp Pattern":dbl[], "y":dbl[]})  [unwired: 1 in]
            }
            frame "3D Gaussian ACF" {
              n137 = Variant To Data(error in=w364, type=T18 {"Amplitude"=0.0, "Diffusion Time"=0.0, "Aspect Ratio"=0.0, "RMSE"=0.0, "R^2"=0.0} ("3D ACF Fit Parameters"), Variant=w366) -> (data=w363:T18, error out=w360:errorcluster)
              n138 = Unbundle By Name(w363) -> ("Aspect Ratio"=w356:dbl, "Amplitude"=w362:dbl, "Diffusion Time"=w361:dbl)
              n139 = formula code="int32 n = sizeOfDim(x,0);\nint32 i;\nfor (i=0; i<n;i++) {\ny[i] = 1+A/(1+x[i]/t)/sqrt(1+x[i]/t/w**2);\n};"("A"=w362, "t"=w361, "x"=w357, "y"=w357, "w"=w356) -> ("y"=w359:dbl[])
              n140 = Bundle("Ramp Pattern"=w357, "y"=w359) -> (w358:cluster{"Ramp Pattern":dbl[], "y":dbl[]})  [unwired: 1 in]
            }
            frame "3D Gaussian + Blinking ACF" {
              n141 = Variant To Data(error in=w378, type=T19 {"Amplitude"=0.0, "Diffusion Time"=0.0, "Aspect Ratio"=0.0, "Blinking Fraction"=0.0, "Blinking Time Constant"=0.0, "RMSE"=0.0, "R^2"=0.0} ("2D Gaussian + Blinking ACF Fit Parameters"), Variant=w379) -> (data=w377:T19, error out=w374:errorcluster)
              n142 = Unbundle By Name(w377) -> ("Amplitude"=w376:dbl, "Diffusion Time"=w375:dbl, "Blinking Fraction"=w370:dbl, "Blinking Time Constant"=w369:dbl, "Aspect Ratio"=w367:dbl)
              n143 = formula code="int32 n = sizeOfDim(x,0);\nint32 i;\nfor (i=0; i<n;i++) {\ny[i] = 1+A/(1+x[i]/t1)/sqrt(1+x[i]/t1/w**2 )*(1-b+b*exp(-x[i]/t2));\n};"("A"=w376, "t1"=w375, "x"=w371, "y"=w371, "b"=w370, "t2"=w369, "w"=w367) -> ("y"=w373:dbl[])
              n144 = Bundle("Ramp Pattern"=w371, "y"=w373) -> (w372:cluster{"Ramp Pattern":dbl[], "y":dbl[]})  [unwired: 1 in]
            }
          }
        }
        frame True {
          # "#todo : residual options"
          n145 = Array Size(array=w383) -> (size(s)=w382:i32)
          n146 = Array Size(array=w384) -> (size(s)=w381:i32)
          n147 = Equal?(x=w382, y=w381) -> (x = y?=w380:bool)
          n148 = case shown="True" w380 {
            tunnel: w386 -> [_ w393]
            tunnel: [_ w392] -> w385
            tunnel: w384 -> [_ w390]
            tunnel: w383 -> [_ w389]
            frame False {
            }
            frame True {
              n149 = Subtract(x=w390, y=w389) -> (x-y=w391:dbl[])
              n150 = Bundle("X Array in"=w393, w391) -> (w392:cluster{"X Array in":dbl[], dbl[]})  [unwired: 1 in]
            }
          }
          n151 = Bundle("X Array in"=w386, "Best Fit in"=w383) -> (w387:cluster{"X Array in":dbl[], "Best Fit in":dbl[]})  [unwired: 1 in]
        }
      }
    }
    frame Error {
      n152 = Bundle("X Array in"=w396, "Best Fit in"=w395) -> (w394:cluster{"X Array in":dbl[], "Best Fit in":dbl[]})  [unwired: 1 in]
    }
  }
  "Error Out" <- w11
  "Array of Component Plots" <- w4
  "Fitted Plot" <- w5
  "Residual Plot" <- w2
